vi "Read Main App Inst Ref.vi"(8 "error in (no error)":errorcluster, 11 "Project in":refnum<class "Project.lvclass">) -> (0 "error out":errorcluster, 2 "Main App Inst Ref":refnum<vi>, 3 "Project out":refnum<class "Project.lvclass">)   [LabVIEW 2020, in "Panther Dashboard.lvlib" / "Project.lvclass"]
uses:
  Project.lvclass
  Project.lvclass/Project.ctl
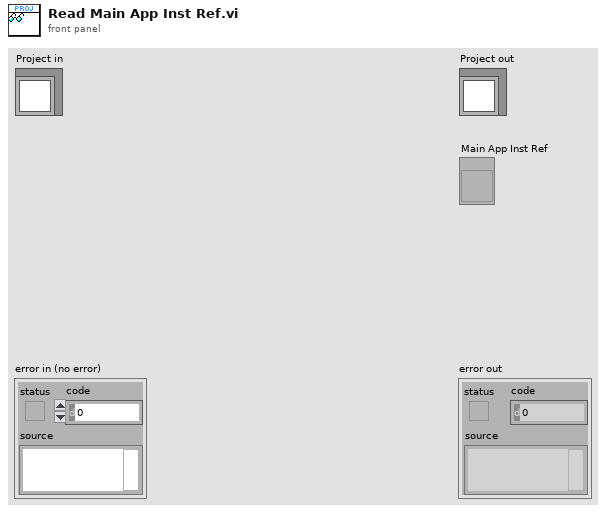
[diagram p1: front panel]
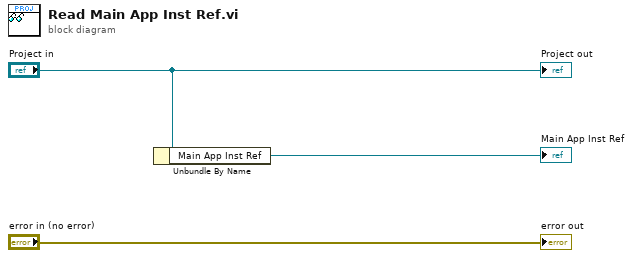
[diagram p0: block diagram]
diagram:
  n1 = Unbundle By Name("Project in") -> ("Main App Inst Ref"=→"Main App Inst Ref":refnum<vi>)
  "error out" <- "error in (no error)"
  "Project out" <- "Project in"
